vi "Result_Test.vi"(8 "error in (no error)":errorcluster caption="entrée d'erreur (pas d'erreur)", 11 "Stop_Ana IN":refnum<class "Stop_Ana.lvclass">) -> (0 "error out":errorcluster caption="sortie d'erreur", 3 "Stop_Ana Out":refnum<class "Stop_Ana.lvclass">)   [LabVIEW 2020, in "Library Test.lvlib" / "Stop_Ana.lvclass"]
uses:
  Stop_Ana.lvclass
  Test_Wtih_Instr/Test_With_Inst.lvclass
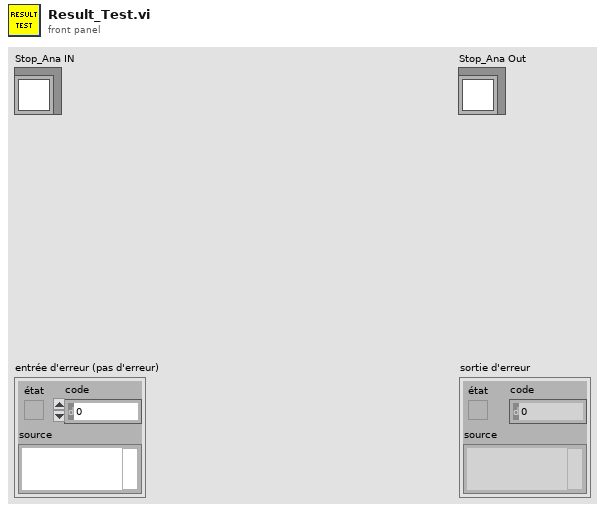
[diagram p1: front panel]
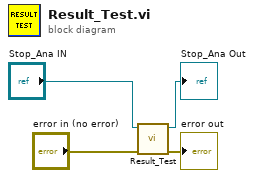
[diagram p0: block diagram]
diagram:
  n1 = call-parent "Result_Test.vi"("error in (no error)"="error in (no error)", "Test_With_Inst en entrée"="Stop_Ana IN") -> ("error out"=→"error out":errorcluster, "Test_With_Inst en sortie"=→"Stop_Ana Out":refnum<class "Stop_Ana.lvclass">)  [unwired: 8 in]
